vi "CSI-2 Tap.vi"(0 "csi-2 input io":T1, 5 "csi-2 output io":T4, 7 "select corrected csi-2 data":bool, 12 "enable tap":bool) -> (4 "serial output channel ready":bool)   [LabVIEW 2020, in "GettingStarted_Acq_Tap_148X_FPGA.lvlib"]
uses:
  GettingStarted_Acq_Tap_148X_FPGA.lvlib
  Common/Types/Serial Output Channel IO.ctl
  Common/Types/Serial Output Channel IO 32b.ctl
  Common/Types/Serial Output Channel IO 64b.ctl
  Types/Serial Input Channel IO.ctl
  Types/Serial Input Channel IO 32b.ctl
  Types/Serial Input Channel IO 64b.ctl
  <vilib>/rvi/eio/common/nirviEmuTemplateMethod_errors.vi
  <vilib>/eio/EIONode/EIONode.xnode
  Common/GettingStarted_Common_148X_FPGA.lvlib
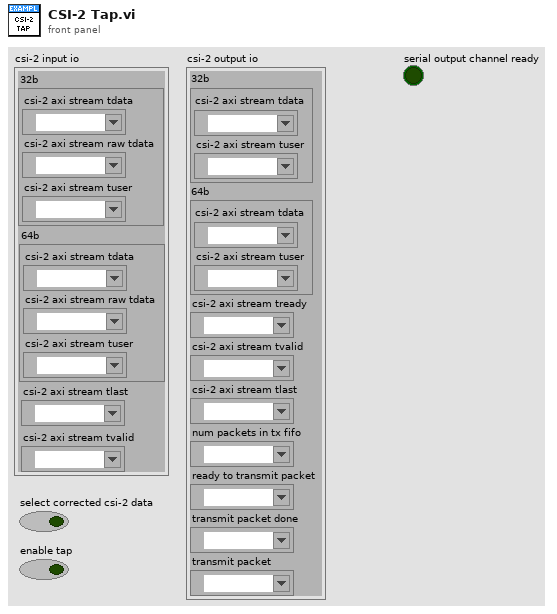
[diagram p1: front panel]
types:
  T1 = typedef "GettingStarted_Acq_Tap_148X_FPGA.lvlib/Serial Input Channel IO.ctl" = cluster{"32b":T2, "64b":T3, "csi-2 axi stream tlast":refnum<k21>, "csi-2 axi stream tvalid":refnum<k21>}
  T2 = typedef "GettingStarted_Acq_Tap_148X_FPGA.lvlib/Serial Input Channel IO 32b.ctl" = cluster{"csi-2 axi stream tdata":refnum<k21>, "csi-2 axi stream raw tdata":refnum<k21>, "csi-2 axi stream tuser":refnum<k21>}
  T3 = typedef "GettingStarted_Acq_Tap_148X_FPGA.lvlib/Serial Input Channel IO 64b.ctl" = cluster{"csi-2 axi stream tdata":refnum<k21>, "csi-2 axi stream raw tdata":refnum<k21>, "csi-2 axi stream tuser":refnum<k21>}
  T4 = typedef "GettingStarted_Common_148X_FPGA.lvlib/Serial Output Channel IO.ctl" = cluster{"32b":T5, "64b":T6, "csi-2 axi stream tready":refnum<k21>, "csi-2 axi stream tvalid":refnum<k21>, "csi-2 axi stream tlast":refnum<k21>, "num packets in tx fifo":refnum<k21>, "ready to transmit packet":refnum<k21>, "transmit packet done":refnum<k21>, "transmit packet":refnum<k21>}
  T5 = typedef "GettingStarted_Common_148X_FPGA.lvlib/Serial Output Channel IO 32b.ctl" = cluster{"csi-2 axi stream tdata":refnum<k21>, "csi-2 axi stream tuser":refnum<k21>}
  T6 = typedef "GettingStarted_Common_148X_FPGA.lvlib/Serial Output Channel IO 64b.ctl" = cluster{"csi-2 axi stream tdata":refnum<k21>, "csi-2 axi stream tuser":refnum<k21>}
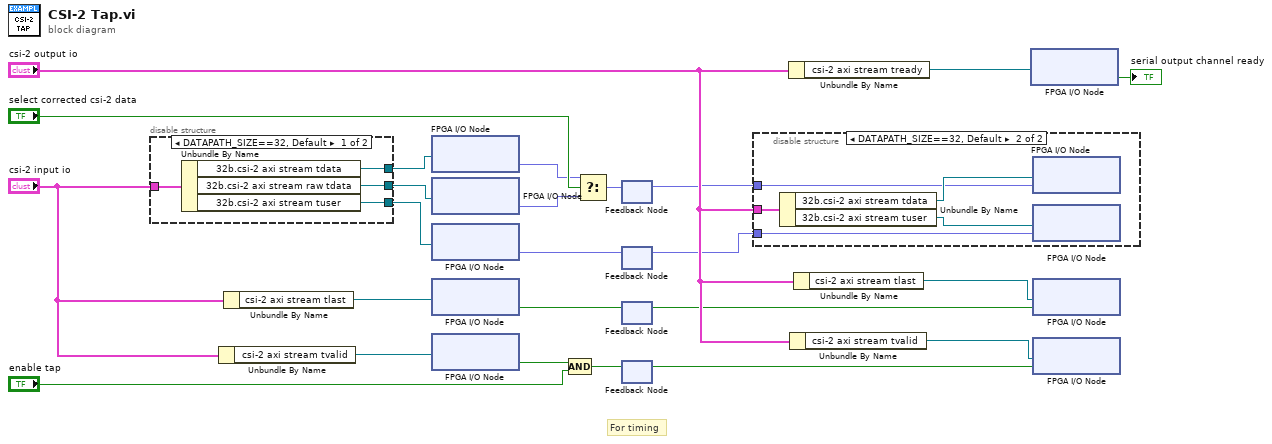
[diagram p0: block diagram]
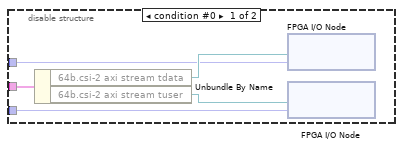
[diagram p2: hidden frame]
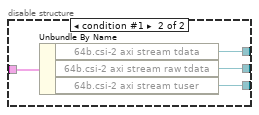
[diagram p3: hidden frame]
diagram:
  # "For timing"
  n1 = disable-structure shown="DATAPATH_SIZE==32, Default" {
    disable-tunnel: "csi-2 input io" -> [w28 w32]
    disable-tunnel: [w25 w29] -> w12
    disable-tunnel: [w27 w31] -> w11
    disable-tunnel: [w26 w30] -> w10
    frame condition #0 (active) {
      n2 = Unbundle By Name(w28) -> ("32b.csi-2 axi stream tdata"=w26:refnum<k21>, "32b.csi-2 axi stream raw tdata"=w27:refnum<k21>, "32b.csi-2 axi stream tuser"=w25:refnum<k21>)
    }
    frame condition #1 {
      n3 = Unbundle By Name(w32) -> ("64b.csi-2 axi stream tdata"=w30:refnum<k21>, "64b.csi-2 axi stream raw tdata"=w31:refnum<k21>, "64b.csi-2 axi stream tuser"=w29:refnum<k21>)
    }
  }
  n4 = Unbundle By Name("csi-2 input io") -> ("csi-2 axi stream tvalid"=w14:refnum<k21>)
  n5 = Unbundle By Name("csi-2 input io") -> ("csi-2 axi stream tlast"=w13:refnum<k21>)
  n6 = xnode "FPGA I/O Node"("FPGA I/O In"=w10) -> ("I/O Item"=w18:fxp<+,32,32>)  [unwired: 1 out]
  n7 = xnode "FPGA I/O Node"("FPGA I/O In"=w11) -> ("I/O Item"=w17:fxp<+,32,32>)  [unwired: 1 out]
  n8 = xnode "FPGA I/O Node"("FPGA I/O In"=w12) -> ("I/O Item"=w5:fxp<+,32,32>)  [unwired: 1 out]
  n9 = xnode "FPGA I/O Node"("FPGA I/O In"=w13) -> ("I/O Item"=w7:bool)  [unwired: 1 out]
  n10 = xnode "FPGA I/O Node"("FPGA I/O In"=w14) -> ("I/O Item"=w23:bool)  [unwired: 1 out]
  n11 = Compound Arithmetic op=AND(w23, "enable tap") -> (w9:bool)
  n12 = Select(t=w18, s="select corrected csi-2 data", f=w17) -> (s? t:f=w4:fxp<+,32,32>)
  n13 = feedback #1() -> (w2:fxp<+,32,32>)  [unwired: 1 in]
  n14 = feedback-in #1(w4) -> ()
  n15 = feedback #2() -> (w1:fxp<+,32,32>)  [unwired: 1 in]
  n16 = feedback-in #2(w5) -> ()
  n17 = feedback #3() -> (w6:bool)  [unwired: 1 in]
  n18 = feedback-in #3(w7) -> ()
  n19 = feedback-in #4(w9) -> ()
  n20 = feedback #4() -> (w8:bool)  [unwired: 1 in]
  n21 = disable-structure shown="DATAPATH_SIZE==32, Default" {
    disable-tunnel: "csi-2 output io" -> [w37 w42]
    disable-tunnel: w2 -> [w34 w39]
    disable-tunnel: w1 -> [w33 w38]
    frame condition #0 {
      n22 = Unbundle By Name(w37) -> ("64b.csi-2 axi stream tdata"=w36:refnum<k21>, "64b.csi-2 axi stream tuser"=w35:refnum<k21>)
      n23 = xnode "FPGA I/O Node"("I/O Item"=w34, "FPGA I/O In"=w36) -> ()  [unwired: 1 out]
      n24 = xnode "FPGA I/O Node"("I/O Item"=w33, "FPGA I/O In"=w35) -> ()  [unwired: 1 out]
    }
    frame condition #1 (active) {
      n25 = Unbundle By Name(w42) -> ("32b.csi-2 axi stream tdata"=w41:refnum<k21>, "32b.csi-2 axi stream tuser"=w40:refnum<k21>)
      n26 = xnode "FPGA I/O Node"("I/O Item"=w39, "FPGA I/O In"=w41) -> ()  [unwired: 1 out]
      n27 = xnode "FPGA I/O Node"("I/O Item"=w38, "FPGA I/O In"=w40) -> ()  [unwired: 1 out]
    }
  }
  n28 = Unbundle By Name("csi-2 output io") -> ("csi-2 axi stream tready"=w21:refnum<k21>)
  n29 = Unbundle By Name("csi-2 output io") -> ("csi-2 axi stream tvalid"=w16:refnum<k21>)
  n30 = Unbundle By Name("csi-2 output io") -> ("csi-2 axi stream tlast"=w15:refnum<k21>)
  n31 = xnode "FPGA I/O Node"("FPGA I/O In"=w21) -> ("I/O Item"=→"serial output channel ready":bool)  [unwired: 1 out]
  n32 = xnode "FPGA I/O Node"("I/O Item"=w6, "FPGA I/O In"=w15) -> ()  [unwired: 1 out]
  n33 = xnode "FPGA I/O Node"("I/O Item"=w8, "FPGA I/O In"=w16) -> ()  [unwired: 1 out]
